vi "DataLog-Update.vi"(0 "state in":T1, 7 "data":dbl[](array[numeric]), 11 "error in (no error)":errorcluster) -> (4 "state out":T1, 15 "error out":errorcluster)   [LabVIEW 2020]
uses:
  DataLog-State.ctl
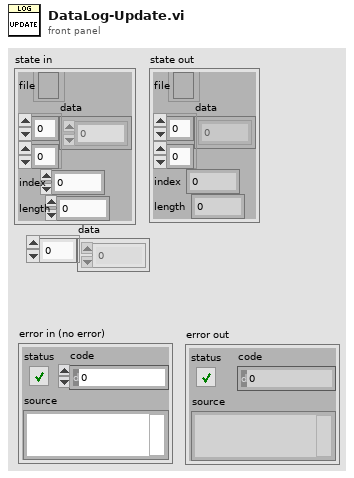
[diagram p1: front panel]
types:
  T1 = typedef "DataLog-State.ctl" = cluster{"file":refnum<file>, "data":dbl[][], "index":i32, "length":i32}
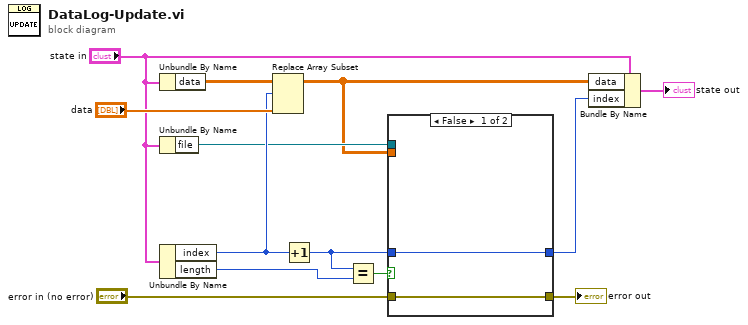
[diagram p0: block diagram]
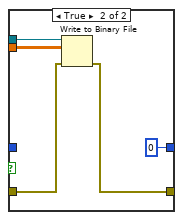
[diagram p2: hidden frame]
diagram:
  n1 = Unbundle By Name("state in") -> ("data"=w13:dbl[][])
  n2 = Unbundle By Name("state in") -> ("file"=w2:refnum<file>)
  n3 = Unbundle By Name("state in") -> ("index"=w11:i32, "length"=w10:i32)
  n4 = Replace Array Subset(array=w13, new element="data", index (row)=w11) -> (w1:dbl[][])  [unwired: 1 in]
  n5 = Increment(x=w11) -> (x+1=w7:i32)
  n6 = Equal?(x=w7, y=w10) -> (x = y?=w9:bool)
  n7 = case shown="False" w9 {
    tunnel: w1 -> [_ w19]
    tunnel: w2 -> [_ w20]
    tunnel: "error in (no error)" -> [w15 w18]
    tunnel: w7 -> [w14 _]
    tunnel: [w15 w16] -> w6
    tunnel: [w14 0] -> w4
    frame False {
    }
    frame True {
      n8 = Write to Binary File(file (use dialog)=w20, data=w19, error in=w18) -> (error out=w16:errorcluster)  [unwired: 3 in, 2 out]
    }
  }
  "error out" <- w6
  n9 = Bundle By Name(cluster="state in", "data"=w1, "index"=w4) -> (→"state out":T1)
